vi "inputfocus_Key.vi"(8 "error in (no error)":errorcluster, 11 "reference":refnum<vi>) -> (0 "error out":errorcluster)   [LabVIEW 2018]
panel:
  in  "String":string
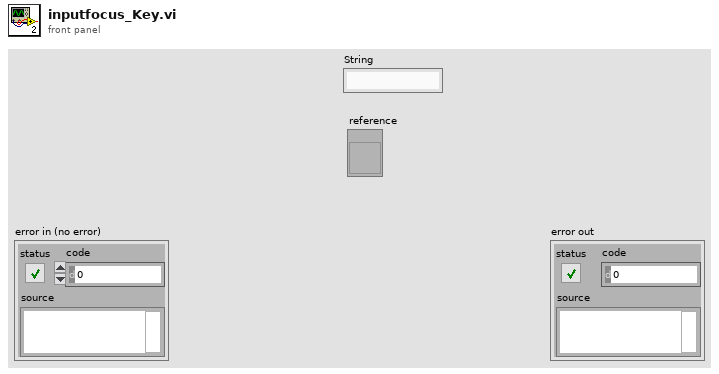
[diagram p1: front panel]
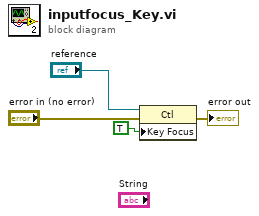
[diagram p0: block diagram]
diagram:
  n1 = property class="Ctl"(reference="reference", error in="error in (no error)", "Key Focus"=TRUE) -> (error out=→"error out":errorcluster)  [unwired: 1 out]
